vi "Auto State Machine.vi"   [LabVIEW 2013]
uses:
  typedefs/fg_typedef.ctl
  <vilib>/Rock Robotics/WPI/Solenoid/WPI_SolenoidValue.ctl
  typedefs/State Machine/singleUseSubstate.ctl
  typedefs/DevRef Type.ctl
  typedefs/State Machine/subStates.ctl
  typedefs/Vision/vision enable.ctl
  <vilib>/Rock Robotics/WPI/Solenoid/WPI_SolenoidSetEnum.vi
panel:
  # "A State Machine to Handle One or Two Ball Autonomous"
types:
  T1 = typedef "fg_typedef.ctl" = enum16{"Get", "Set"}
  T2 = typedef "WPI_SolenoidValue.ctl" = enum16{"Off", "On", "Forward", "Reverse"}
  T3 = typedef "singleUseSubstate.ctl" = enum16{"null", "wait", "shift high", "shift low", "extend shooter", "retract shooter", "latch", "unlatch", "end"}
  T4 = typedef "subStates.ctl" = enum16{"null", "wait", "driver control", "auto", "manual override", "hold position", "rotate", "pickup", "pass", "recover pass", "load", "goto shoot", "shoot high goal", "shoot low goal", "cancel arm", "cancel shooter", "end", "test"}
  T5 = typedef "vision enable.ctl" = enum16{"Enable", "Disable", "Stop"}
  T6 = typedef "DevRef Type.ctl" = enum16{"Shooter Solenoid", "Latch Solenoid", "Right Up Sensor", "Right Down Sensor", "Hold Sensor", "Arm Encoder"}
  T7 = typedef "WPI_EncoderDevRef.ctl" = cluster{"DevStatus":errorcluster, "EncoderIndex":T8, "CounterIndex":T9, "DistancePerCount":dbl, "Decoding Type":T10}
  T8 = typedef "FPGA_EncoderIdx.ctl" = enum8{"Enc 0", "Enc 1", "Enc 2", "Enc 3", "Invalid"}
  T9 = typedef "FPGA_CounterCtrSystemIndex.ctl" = enum8{"Ctr 0", "Ctr 1", "Ctr 2", "Ctr 3", "Ctr 4", "Ctr 5", "Ctr 6", "Ctr 7", "Invalid"}
  T10 = typedef "WPI_EncoderType.ctl" = enum16{"1x", "2x", "4x"}
  T11 = typedef "WPI_SolenoidDevRef.ctl" = cluster{"DevStatus":errorcluster, "Solenoid Module":T12, "Forward Solenoid Channel":T13, "Reverse Solenoid Channel":T13}
  T12 = typedef "FPGA_TypedefSolenoidModule.ctl" = enum16{"Solenoid Module 1", "Solenoid Module 2"}
  T13 = typedef "WPI_SolenoidChannel.ctl" = enum8{"Solenoid 1", "Solenoid 2", "Solenoid 3", "Solenoid 4", "Solenoid 5", "Solenoid 6", "Solenoid 7", "Solenoid 8", "Invalid"}
  T14 = typedef "WPI_DigitalInputDevRef.ctl" = cluster{"DevStatus":errorcluster, "DIO Channel":T15, "Digital Module":T16}
  T15 = typedef "FPGA_DIOChannel.ctl" = enum8{"DIO 1", "DIO 2", "DIO 3", "DIO 4", "DIO 5", "DIO 6", "DIO 7", "DIO 8", "DIO 9", "DIO 10", "DIO 11", "DIO 12", "DIO 13", "DIO 14", "Invalid"}
  T16 = typedef "FPGA_TypedefDigitalModule.ctl" = enum16{"Digital Module 1", "Digital Module 2"}
  T17 = typedef "vision data.ctl" = cluster{"x":dbl, "y":dbl, "area":dbl, "width":dbl, "height":dbl, "Hot Goal Present?":bool, "distance":dbl}
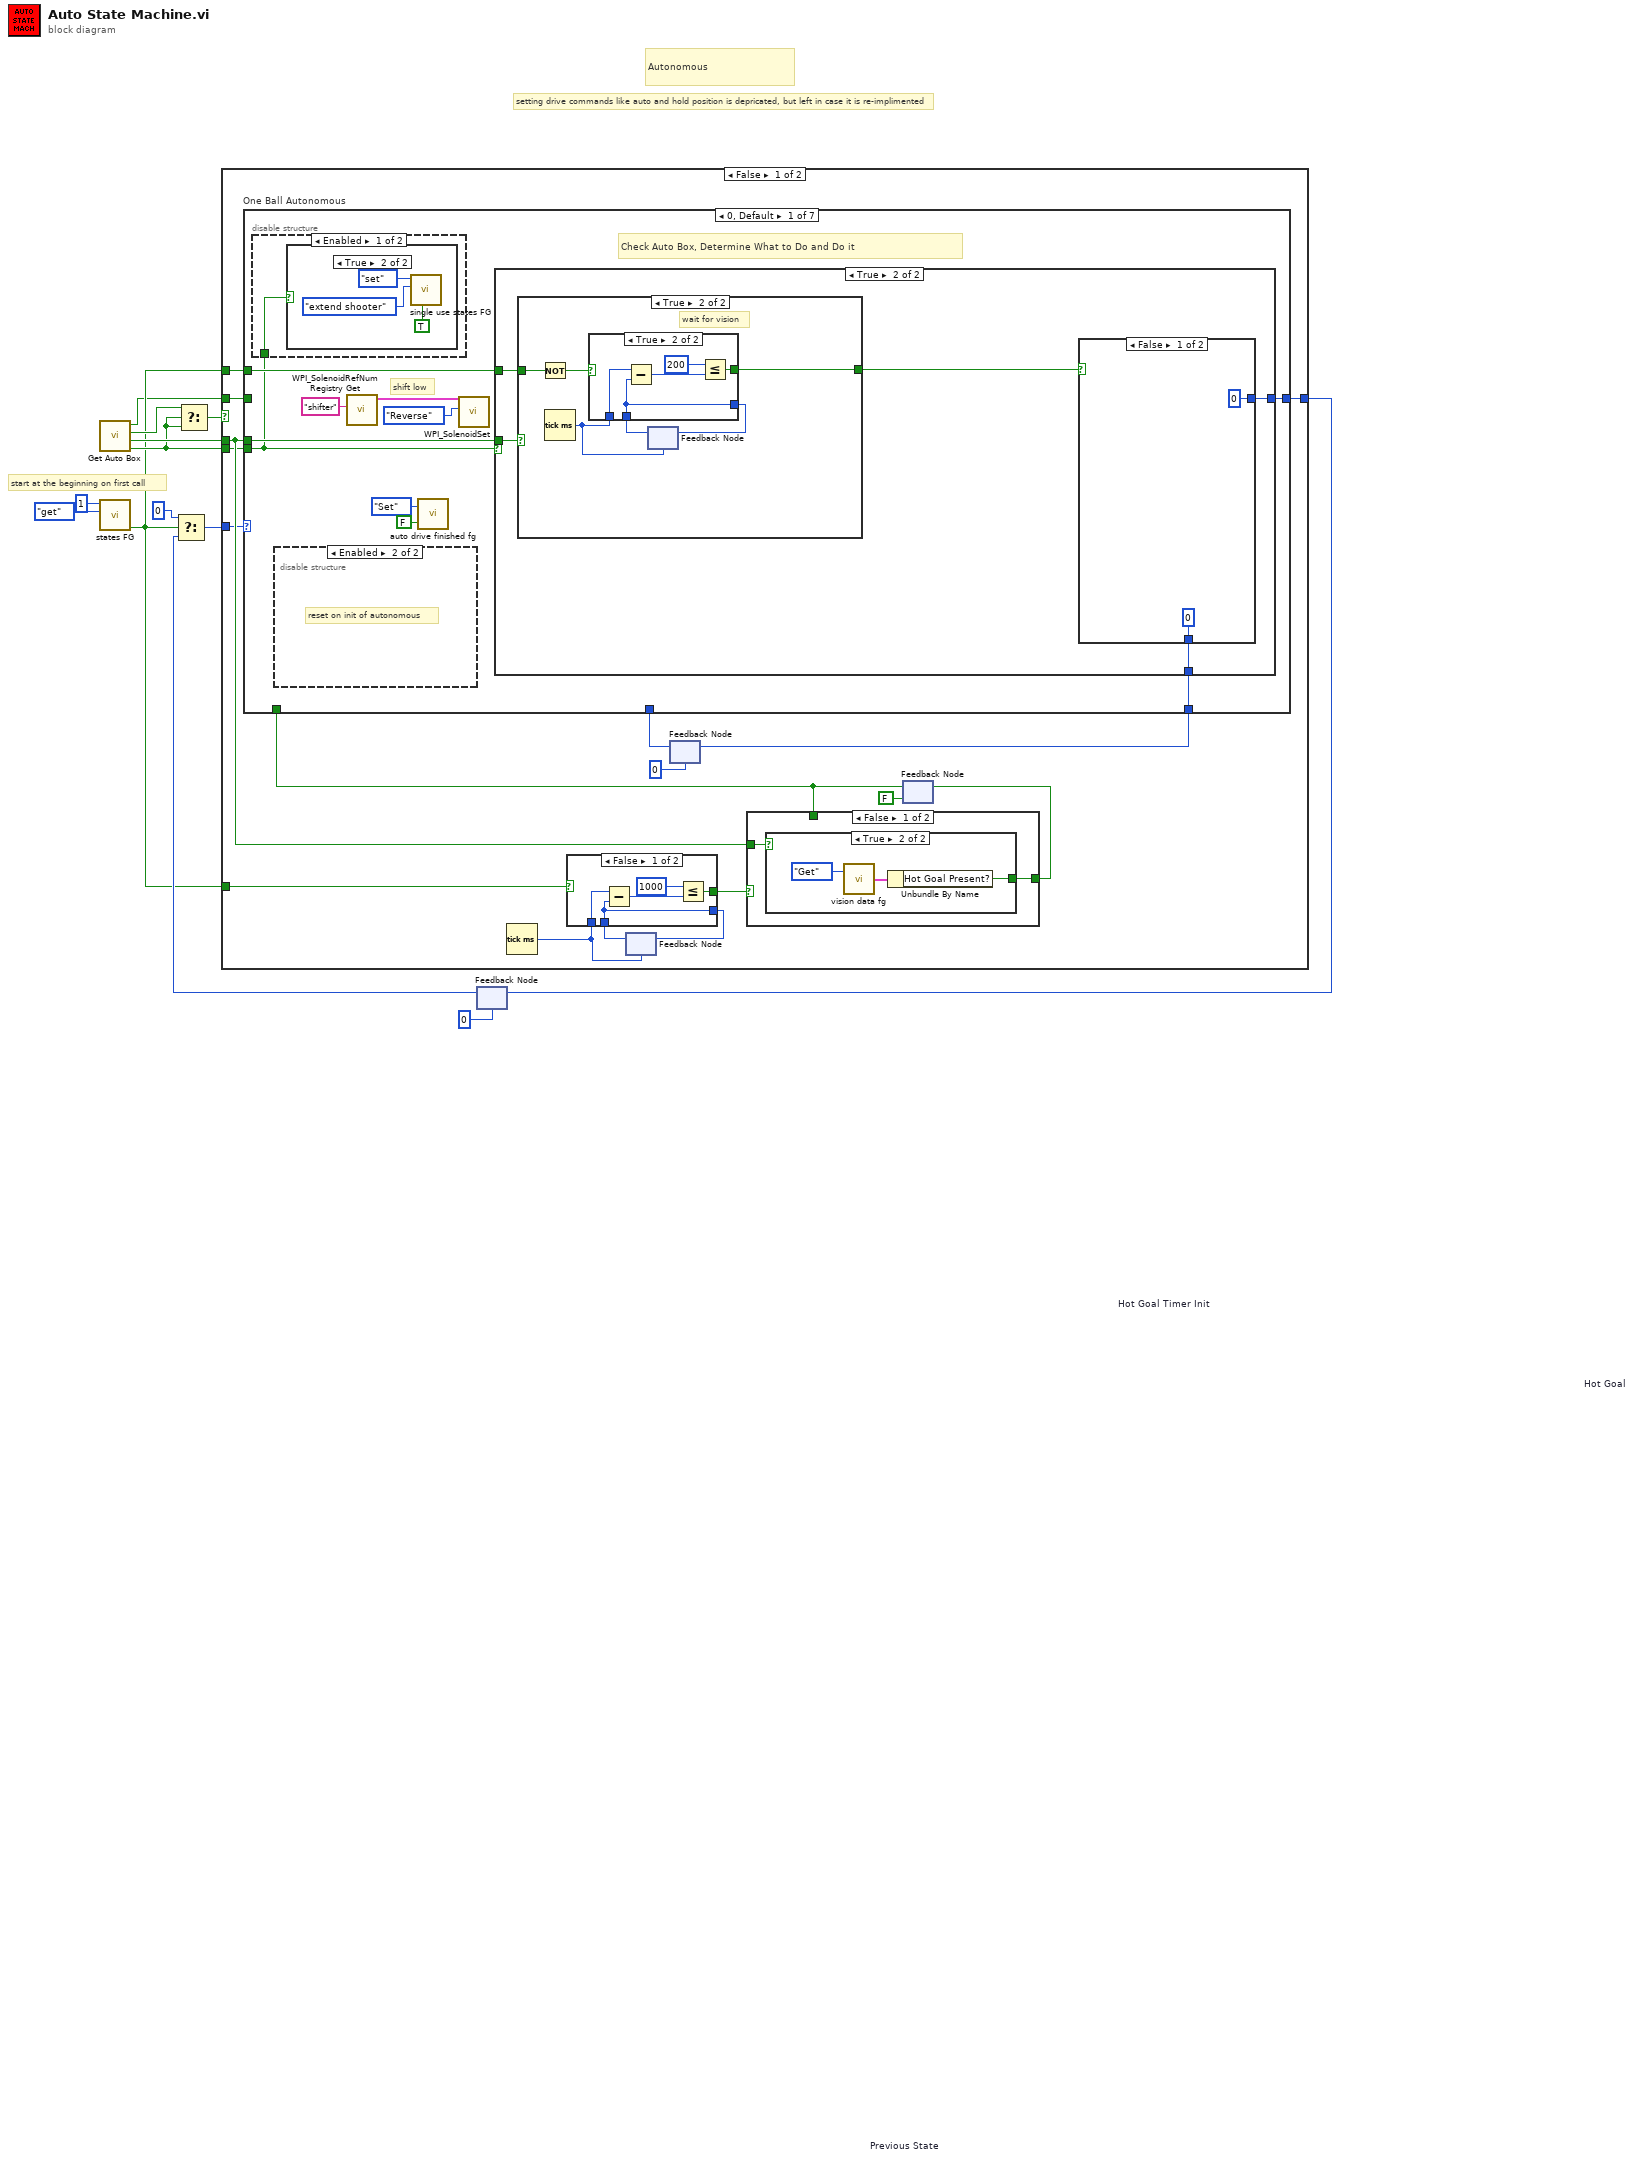
[diagram p0: block diagram]
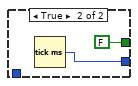
[diagram p2: hidden frame]
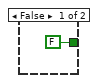
[diagram p3: hidden frame]
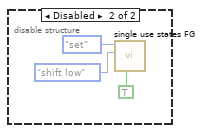
[diagram p6: hidden frame]
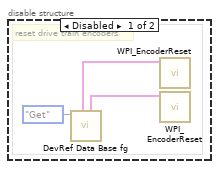
[diagram p7: hidden frame]
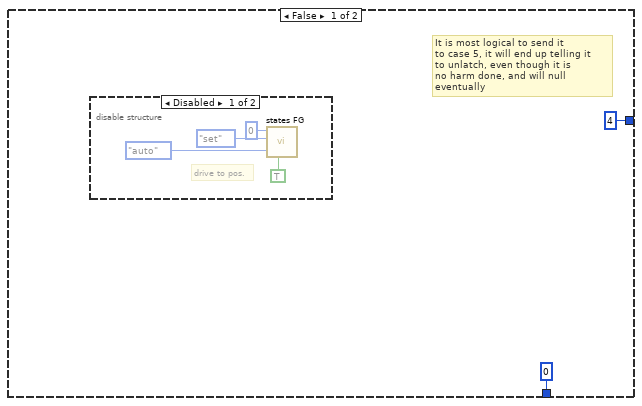
[diagram p8: hidden frame]
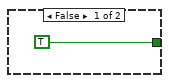
[diagram p10: hidden frame]
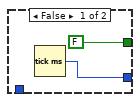
[diagram p11: hidden frame]
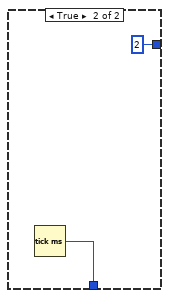
[diagram p12: hidden frame]
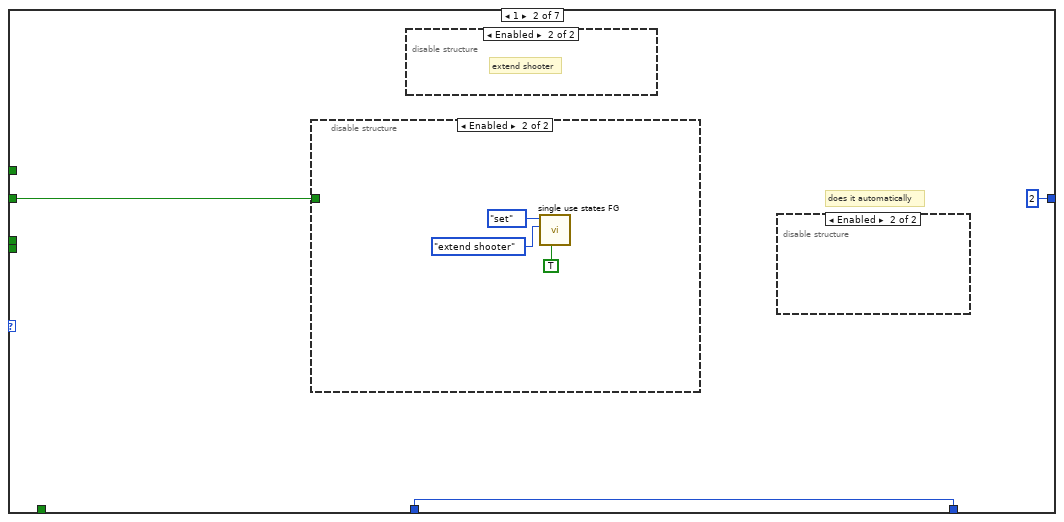
[diagram p13: hidden frame]
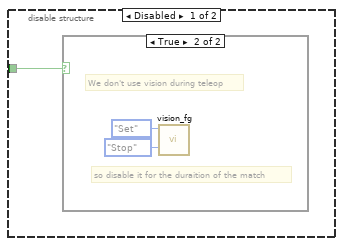
[diagram p15: hidden frame]
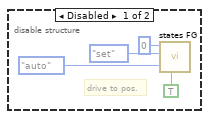
[diagram p17: hidden frame]
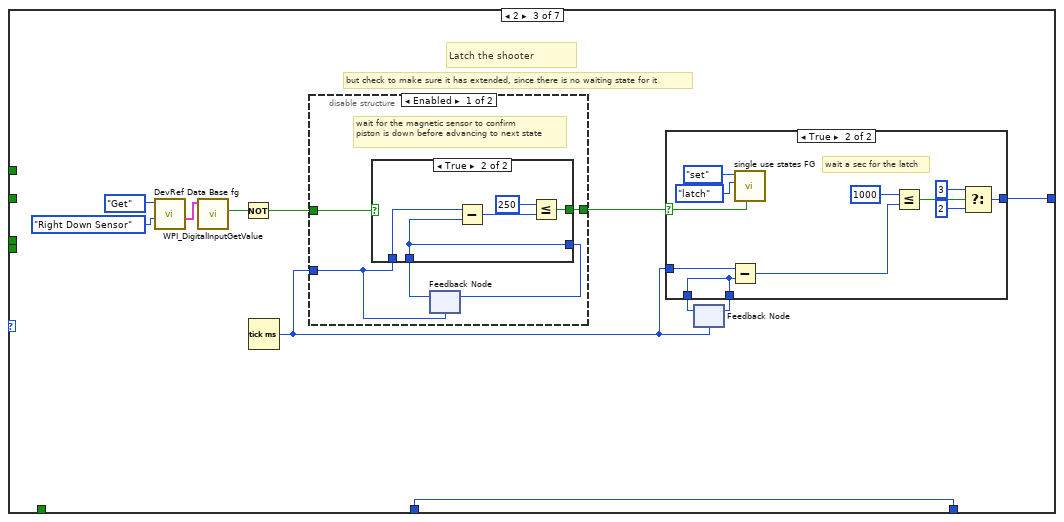
[diagram p18: hidden frame]
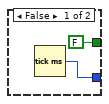
[diagram p19: hidden frame]
diagram:
  # "setting drive commands like auto and hold position is depricated, but left in case it is re-implimented"
  # "start at the beginning on first call"
  # "Autonomous"
  n1 = call "Get Auto Box.vi"() -> ("Shoot During Autonomous?"=w3:bool, "Use Hot Goal?"=w6:bool, "2 Ball Autonomous?"=w4:bool, "Disable Vison After Auto?"=w1:bool)
  n2 = call "states FG.vi"("menu (get)"=enum16{"set", "get"}."get", "Loop ID"=1) -> ("first call?"=w2:bool)  [unwired: 6 in, 3 out]
  n3 = Select(t=w4, s=w3, f=w3) -> (s? t:f=w5:bool)
  n4 = feedback #1 "Previous State"(u8 0) -> (w9:u8)
  n5 = Select(t=u8 0, s=w2, f=w9) -> (s? t:f=w11:u8)
  n6 = case shown="False" w5 {
    tunnel: w11 -> [w29 w236]
    tunnel: [w28 w229] -> w7
    tunnel: w2 -> [w26 w225]
    tunnel: w3 -> [w25 _]
    tunnel: w6 -> [w30 _]
    tunnel: w2 -> [w17 w233]
    tunnel: w1 -> [w23 _]
    frame False {
      n7 = Tick Count (ms)() -> (millisecond timer value=w15:u32)
      n8 = feedback #2(w15) -> (w20:u32)
      n9 = case shown="False" w17 {
        tunnel: [w32 w37] -> w19
        tunnel: w20 -> [w32 _]
        tunnel: [w33 FALSE] -> w18
        tunnel: w15 -> [w31 _]
        frame False {
          n10 = Subtract(x=w31, y=w32) -> (x-y=w35:u32)
          n11 = Less Or Equal?(x=u32 1000, y=w35) -> (x <= y?=w33:bool)
        }
        frame True {
          n12 = Tick Count (ms)() -> (millisecond timer value=w37:u32)
        }
      }
      n13 = feedback-in #2(w19) -> ()
      n14 = feedback #3 "Hot Goal Timer Init"(u32 0 ("millisecond timer value")) -> (w16:u32)
      n15 = feedback #4 "Hot Goal"(FALSE ("Hot Goal Present?")) -> (w14:bool)
      n16 = case "One Ball Autonomous" shown="0, Default" w29 {
        selector: w29 -> [_ _ _ _ w163 _ w222]
        tunnel: [w54 u8 2 ("t") w113 u8 4 ("t") w161 u8 6 ("t") w222] -> w28
        tunnel: w16 -> [_ w96 w107 w144 w151 w197 w205]
        tunnel: w26 -> [w53 _ _ _ _ _ _]
        tunnel: w25 -> [w51 _ _ _ w154 _ _]
        tunnel: w30 -> [w52 _ _ _ _ _ _]
        tunnel: [w50 w96 w107 w144 w151 w197 w205] -> w24
        tunnel: w23 -> [_ w94 _ _ _ _ w204]
        tunnel: w14 -> [_ _ _ _ w153 _ _]
        frame 0, Default {
          # "shift low"
          # "Check Auto Box, Determine What to Do and Do it"
          n17 = disable-structure shown="Enabled" {
            disable-tunnel: w51 -> [w55 _]
            frame Enabled {
              n18 = case shown="True" w55 {
                frame False {
                }
                frame True {
                  n19 = call "single use states FG.vi"("exit in"=TRUE, "substate"=singleUseSubstate."extend shooter", "menu (get)"=enum16{"set", "get"}."set") -> ()  [unwired: 5 in, 4 out]
                }
              }
            }
            frame Disabled {
              n20 = call "single use states FG.vi"("exit in"=TRUE, "substate"=singleUseSubstate."shift low", "menu (get)"=enum16{"set", "get"}."set") -> ()  [unwired: 5 in, 4 out]
            }
          }
          n21 = disable-structure shown="Enabled" {
            frame Disabled {
              # "reset drive train encoders"
              n22 = call "DevRef Data Base fg.vi"("Menu"=fg_typedef."Get") -> ("right drive encoder"=w62:T7, "left drive encoder"=w63:T7)  [unwired: 2 in, 7 out]
              n23 = call <vilib>:"WPI_EncoderReset.vi"("EncoderDevRef"=w63) -> ()  [unwired: 9 in, 2 out]
              n24 = call <vilib>:"WPI_EncoderReset.vi"("EncoderDevRef"=w62) -> ()  [unwired: 9 in, 2 out]
            }
            frame Enabled {
              # "reset on init of autonomous"
            }
          }
          n25 = call <vilib>:"WPI_SolenoidRefNum Registry Get.vi"("refnum name"="shifter") -> ("SolenoidDevRef"=w45:T11)  [unwired: 9 in, 1 out]
          n26 = call "auto drive finished fg.vi"("Done?"=FALSE, "Menu"=fg_typedef."Set") -> ()  [unwired: 1 out]
          n27 = call-poly <vilib>:"WPI_SolenoidSet.vi"("Value"=WPI_SolenoidValue."Reverse", "SolenoidDevRef"=w45) -> ()  [unwired: 8 in, 2 out]
          n28 = case shown="True" w51 {
            tunnel: [u8 4 ("f") w75] -> w54
            tunnel: w53 -> [_ w74]
            tunnel: w52 -> [_ w72]
            tunnel: [u32 0 ("millisecond timer value") w71] -> w50
            frame False {
              # "It is most logical to send it\nto case 5, it will end up telling it\nto unlatch, even though it is\nno harm done, and will null eventually"
              n29 = disable-structure shown="Disabled" {
                frame Disabled {
                  # "drive to pos."
                  n30 = call "states FG.vi"("exit in"=TRUE, "subState in"=subStates."auto", "menu (get)"=enum16{"set", "get"}."set", "Loop ID"=0) -> ()  [unwired: 4 in, 4 out]
                }
                frame Enabled {
                }
              }
            }
            frame True {
              n31 = case shown="True" w72 {
                tunnel: w74 -> [_ w82]
                tunnel: [TRUE w81] -> w73
                frame False {
                }
                frame True {
                  # "wait for vision"
                  n32 = Not(x=w82) -> (.not. x?=w77:bool)
                  n33 = Tick Count (ms)() -> (millisecond timer value=w80:u32)
                  n34 = feedback #5(w80) -> (w78:u32)
                  n35 = case shown="True" w77 {
                    tunnel: w80 -> [_ w87]
                    tunnel: [w84 w85] -> w79
                    tunnel: w78 -> [_ w85]
                    tunnel: [FALSE w86] -> w81
                    frame False {
                      n36 = Tick Count (ms)() -> (millisecond timer value=w84:u32)
                    }
                    frame True {
                      n37 = Subtract(x=w87, y=w85) -> (x-y=w89:u32)
                      n38 = Less Or Equal?(x=u32 200, y=w89) -> (x <= y?=w86:bool)
                    }
                  }
                  n39 = feedback-in #5(w79) -> ()
                }
              }
              n40 = case shown="False" w73 {
                tunnel: [u8 0 ("f") u8 2 ("f")] -> w75
                tunnel: [u32 0 ("millisecond timer value") w92] -> w71
                frame False {
                }
                frame True {
                  n41 = Tick Count (ms)() -> (millisecond timer value=w92:u32)
                }
              }
            }
          }
        }
        frame 1 {
          # "does it automatically"
          n42 = disable-structure shown="Enabled" {
            disable-tunnel: w94 -> [w97 _]
            frame Disabled {
              n43 = case shown="True" w97 {
                frame False {
                }
                frame True {
                  # "so disable it for the duraition of the match"
                  # "We don't use vision during teleop"
                  n44 = call "vision_fg.vi"("Action"=vision_enable."Stop", "Menu"=fg_typedef."Set" ("Enum")) -> ()  [unwired: 1 in, 2 out]
                }
              }
            }
            frame Enabled {
              n45 = call "single use states FG.vi"("exit in"=TRUE, "substate"=singleUseSubstate."extend shooter", "menu (get)"=enum16{"set", "get"}."set") -> ()  [unwired: 5 in, 4 out]
            }
          }
          n46 = disable-structure shown="Enabled" {
            frame Disabled {
              # "this has become completly unused now"
              # "Drive Up"
            }
            frame Enabled {
              # "extend shooter"
            }
          }
          n47 = disable-structure shown="Enabled" {
            frame Disabled {
              # "drive to pos."
              n48 = call "states FG.vi"("exit in"=TRUE, "subState in"=subStates."auto", "menu (get)"=enum16{"set", "get"}."set", "Loop ID"=0) -> ()  [unwired: 4 in, 4 out]
            }
            frame Enabled {
            }
          }
        }
        frame 2 {
          # "but check to make sure it has extended, since there is no waiting state for it"
          # "Latch the shooter"
          n49 = call "DevRef Data Base fg.vi"("DevRef to Get"=DevRef_Type."Right Down Sensor", "Menu"=fg_typedef."Get") -> ("Selected Sensor"=w117:T14)  [unwired: 1 in, 8 out]
          n50 = call <vilib>:"WPI_DigitalInputGetValue.vi"("DigitalInputDevRef"=w117) -> ("Value"=w116:bool)  [unwired: 8 in, 2 out]
          n51 = Not(x=w116) -> (.not. x?=w110:bool)
          n52 = Tick Count (ms)() -> (millisecond timer value=w109:u32)
          n53 = disable-structure shown="Enabled" {
            disable-tunnel: w110 -> [w122 w130]
            disable-tunnel: [w119 w130] -> w108
            disable-tunnel: w109 -> [w118 _]
            frame Enabled {
              # "wait for the magnetic sensor to confirm \npiston is down before advancing to next state"
              n54 = feedback #6(w118) -> (w120:u32)
              n55 = case shown="True" w122 {
                tunnel: w118 -> [_ w127]
                tunnel: [w124 w125] -> w121
                tunnel: w120 -> [_ w125]
                tunnel: [FALSE w126] -> w119
                frame False {
                  n56 = Tick Count (ms)() -> (millisecond timer value=w124:u32)
                }
                frame True {
                  n57 = Subtract(x=w127, y=w125) -> (x-y=w129:u32)
                  n58 = Less Or Equal?(x=u32 250, y=w129) -> (x <= y?=w126:bool)
                }
              }
              n59 = feedback-in #6(w121) -> ()
            }
            frame Disabled {
            }
          }
          n60 = feedback #7(w109) -> (w114:u32)
          n61 = case shown="True" w108 {
            selector: w108 -> [_ w139]
            tunnel: [w131 w141] -> w115
            tunnel: w114 -> [_ w141]
            tunnel: w109 -> [w131 w140]
            tunnel: [u8 2 ("f") w134] -> w113
            frame False {
              # "wait for the shooter"
            }
            frame True {
              # "wait a sec for the latch"
              n62 = Subtract(x=w140, y=w141) -> (x-y=w136:u32)
              n63 = call "single use states FG.vi"("exit in"=w139, "substate"=singleUseSubstate."latch", "menu (get)"=enum16{"set", "get"}."set") -> ()  [unwired: 5 in, 4 out]
              n64 = Less Or Equal?(x=u32 1000, y=w136) -> (x <= y?=w133:bool)
              n65 = Select(t=u8 3, s=w133, f=u8 2) -> (s? t:f=w134:u8)
            }
          }
          n66 = feedback-in #7(w115) -> ()
        }
        frame 3 {
          # "just go on, nothing to\nwait for"
          # "retract shooter"
          n67 = call "single use states FG.vi"("exit in"=TRUE, "substate"=singleUseSubstate."retract shooter", "menu (get)"=enum16{"set", "get"}."set") -> ()  [unwired: 5 in, 4 out]
        }
        frame 4 {
          # "depends on if shooting"
          # "at setpoint?"
          n68 = case shown="False" w153 {
            tunnel: w151 -> [w180 w186]
            tunnel: [w179 w185] -> w152
            frame True {
              # "get it first cycle after 3.5 seconds"
              n69 = Tick Count (ms)() -> (millisecond timer value=w181:u32)
              n70 = Subtract(x=w181, y=w180) -> (x-y=w183:u32)
              n71 = disable-structure shown="Disabled" {
                disable-tunnel: [_ FALSE ("Done")] -> w177
                frame Disabled {
                }
                frame Enabled {
                }
              }
              n72 = Less Or Equal?(x=u32 3500, y=w183) -> (x <= y?=w178:bool)
              n73 = Or(x=w178, y=w177) -> (x .or. y?=w179:bool)
            }
            frame False {
              # "wait 5.25 seconds for hot goal to switch"
              n74 = Tick Count (ms)() -> (millisecond timer value=w187:u32)
              n75 = Subtract(x=w187, y=w186) -> (x-y=w189:u32)
              n76 = Less Or Equal?(x=u32 5250, y=w189) -> (x <= y?=w185:bool)
            }
          }
          n77 = disable-structure shown="Enabled" {
            disable-tunnel: w151 -> [w166 _]
            frame Disabled {
              n78 = Tick Count (ms)() -> (millisecond timer value=w169:u32)
              n79 = Subtract(x=w169, y=w166) -> (x-y=w167:u32)
              n80 = Less Or Equal?(x=u32 4100, y=w167) -> (x <= y?=w165:bool)
              n81 = disable-structure shown="Enabled" {
                disable-tunnel: w165 -> [w171 _]
                disable-tunnel: fg_typedef."Set" ("Menu") -> [w170 _]
                frame Enabled {
                  n82 = case shown="True" w171 {
                    selector: w171 -> [_ w173]
                    tunnel: w170 -> [_ w172]
                    frame False {
                    }
                    frame True {
                      n83 = call "auto drive finished fg.vi"("Done?"=w173, "Menu"=w172) -> ()  [unwired: 1 out]
                      n84 = call "states FG.vi"("exit in"=w173, "subState in"=subStates."null" ("y"), "menu (get)"=enum16{"set", "get"}."set", "Loop ID"=0) -> ()  [unwired: 4 in, 4 out]
                    }
                  }
                }
                frame Disabled {
                }
              }
            }
            frame Enabled {
            }
          }
          n85 = call "DevRef Data Base fg.vi"("DevRef to Get"=DevRef_Type."Right Up Sensor", "Menu"=fg_typedef."Get") -> ("Selected Sensor"=w160:T14)  [unwired: 1 in, 8 out]
          n86 = call <vilib>:"WPI_DigitalInputGetValue.vi"("DigitalInputDevRef"=w160) -> ("Value"=w159:bool)  [unwired: 8 in, 2 out]
          n87 = Not(x=w159) -> (.not. x?=w156:bool)
          n88 = case shown="True" w156 {
            frame False {
            }
            frame True {
              # "incase we have problems,\nlet drivers trigger shoot after auto\nsince it is infact safe to shoot now"
              n89 = call "safe shoot error.vi"("Can Shoot Safely?"=TRUE, "Menu"=fg_typedef."Set") -> ()  [unwired: 1 out]
            }
          }
          n90 = call "auto drive finished fg.vi"("Menu"=fg_typedef."Get") -> ("Done"=w149:bool)  [unwired: 1 in]
          n91 = case shown="False" w154 {
            tunnel: w152 -> [_ w194]
            tunnel: w156 -> [_ w193]
            tunnel: w149 -> [w190 w192]
            tunnel: [w190 w191] -> w155
            frame False {
            }
            frame True {
              n92 = Compound Arithmetic op=AND(w194, w193, w192) -> (w191:bool)
            }
          }
          n93 = Select(t=u8 5, s=w155, f=w163) -> (s? t:f=w161:u8)
        }
        frame 5 {
          w200 = FALSE ("Can Shoot Safely?")
          w199 = fg_typedef."Set" ("Menu")
          # "unlatch shooter"
          # "SHOOT!!!"
          n94 = call "safe shoot error.vi"("Can Shoot Safely?"=w200, "Menu"=w199) -> ()  [unwired: 1 out]
          n95 = call "auto drive finished fg.vi"("Done?"=w200, "Menu"=w199) -> ()  [unwired: 1 out]
          n96 = call "single use states FG.vi"("exit in"=TRUE, "substate"=singleUseSubstate."unlatch", "menu (get)"=enum16{"set", "get"}."set") -> ()  [unwired: 5 in, 4 out]
        }
        frame 6 {
          # "null things"
          # "null all the things"
          n97 = case shown="True" w204 {
            frame False {
            }
            frame True {
              # "so disable it for the duraition of the match"
              # "We don't use vision during teleop"
              n98 = call "vision_fg.vi"("Action"=vision_enable."Stop", "Menu"=fg_typedef."Set" ("Enum")) -> ()  [unwired: 1 in, 2 out]
            }
          }
          n99 = call "states FG.vi"("exit in"=TRUE, "subState in"=subStates."null", "menu (get)"=enum16{"set", "get"}."set", "Loop ID"=0) -> ()  [unwired: 4 in, 4 out]
          n100 = call "states FG.vi"("exit in"=TRUE, "subState in"=subStates."null", "menu (get)"=enum16{"set", "get"}."set", "Loop ID"=1) -> ()  [unwired: 4 in, 4 out]
          n101 = call "states FG.vi"("exit in"=TRUE, "subState in"=subStates."null", "menu (get)"=enum16{"set", "get"}."set", "Loop ID"=2) -> ()  [unwired: 4 in, 4 out]
          n102 = call "states FG.vi"("exit in"=TRUE, "subState in"=subStates."null", "menu (get)"=enum16{"set", "get"}."set", "Loop ID"=3) -> ()  [unwired: 4 in, 4 out]
        }
      }
      n103 = feedback-in #3(w24) -> ()
      n104 = case shown="False" w18 {
        tunnel: [w39 w44] -> w21
        tunnel: w14 -> [_ w44]
        tunnel: w30 -> [w38 _]
        frame False {
          n105 = case shown="True" w38 {
            tunnel: [FALSE ("Hot Goal Present?") w43] -> w39
            frame False {
            }
            frame True {
              n106 = call "vision data fg.vi"("Menu"=fg_typedef."Get") -> ("Output"=w42:T17)  [unwired: 1 in]
              n107 = Unbundle By Name(w42) -> ("Hot Goal Present?"=w43:bool)
            }
          }
        }
        frame True {
        }
      }
      n108 = feedback-in #4(w21) -> ()
    }
    frame True {
      n109 = feedback #8 "Wait Timer Init"(u32 0 ("millisecond timer value")) -> (w226:u32)
      n110 = case "Two Ball Autonomous" shown="0, Default" w236 {
        selector: w236 -> [_ w313 _ w332 _ w366 _ _ w387 w425 _ w443]
        tunnel: [u8 1 ("t") w315 u8 3 ("t") w329 u8 5 ("t") w368 u8 7 ("t") u8 8 ("t") w388 w424 u8 11 ("t") w443] -> w229
        tunnel: [_ _ w323 w330 _ _ _ _ _ _ _ _] -> w227
        tunnel: w226 -> [_ _ _ w331 _ _ _ _ _ _ _ _]
        tunnel: w225 -> [w294 _ _ _ _ _ _ _ _ _ _ _]
        frame 0, Default {
          # "full reverse is belts in"
          # "belts on"
          # "up setpoint"
          # "put arm out"
          # "Arm Up, Belts In"
          # "reset drive train encoders"
          n111 = case shown="True" w294 {
            frame False {
            }
            frame True {
              # "so disable it for the duraition of the match"
              # "We don't use vision during teleop"
              n112 = call "vision_fg.vi"("Action"=vision_enable."Stop", "Menu"=fg_typedef."Set" ("Enum")) -> ()  [unwired: 1 in, 2 out]
            }
          }
          n113 = call "auto drive finished fg.vi"("Done?"=FALSE, "Menu"=fg_typedef."Set") -> ()  [unwired: 1 out]
          n114 = call "Arm Setpoint FG.vi"("Setpoint In"=55.0, "Menu"=fg_typedef."Set") -> ()  [unwired: 1 out]
          n115 = call "states FG.vi"("exit in"=TRUE, "subState in"=subStates."auto", "menu (get)"=enum16{"set", "get"}."set", "Loop ID"=3) -> ()  [unwired: 4 in, 4 out]
          n116 = call "Belt Speed FG.vi"("Speed In"=-1.0 ("Setpoint In"), "Menu"=fg_typedef."Set") -> ()  [unwired: 1 out]
          n117 = call "states FG.vi"("exit in"=TRUE, "subState in"=subStates."auto", "menu (get)"=enum16{"set", "get"}."set", "Loop ID"=2) -> ()  [unwired: 4 in, 4 out]
          n118 = call "DevRef Data Base fg.vi"("Menu"=fg_typedef."Get") -> ("right drive encoder"=w308:T7, "left drive encoder"=w309:T7)  [unwired: 2 in, 7 out]
          n119 = call <vilib>:"WPI_EncoderReset.vi"("EncoderDevRef"=w309) -> ()  [unwired: 9 in, 2 out]
          n120 = call <vilib>:"WPI_EncoderReset.vi"("EncoderDevRef"=w308) -> ()  [unwired: 9 in, 2 out]
        }
        frame 1 {
          # "Wait for Arm"
          n121 = call "DevRef Data Base fg.vi"("DevRef to Get"=DevRef_Type."Arm Encoder", "Menu"=fg_typedef."Get") -> ("Selected Encoder"=w322:T7)  [unwired: 1 in, 8 out]
          n122 = call <vilib>:"WPI_EncoderGet.vi"("EncoderDevRef"=w322) -> ("Distance"=w321:dbl)  [unwired: 5 in, 5 out]
          n123 = In Range and Coerce(upper limit=55.0, x=w321, lower limit=45.0) -> (In Range?=w314:bool)  [unwired: 1 out]
          n124 = Select(t=u8 2, s=w314, f=w313) -> (s? t:f=w315:u8)
        }
        frame 2 {
          # "drive to reverse position"
          n125 = Tick Count (ms)() -> (millisecond timer value=w323:u32)
          n126 = call "states FG.vi"("exit in"=TRUE, "subState in"=subStates."auto", "menu (get)"=enum16{"set", "get"}."set", "Loop ID"=0) -> ()  [unwired: 4 in, 4 out]
        }
        frame 3 {
          # "Wait for Ball"
          n127 = disable-structure shown="Enabled" {
            disable-tunnel: w332 -> [w334 w343]
            disable-tunnel: w331 -> [_ w345]
            disable-tunnel: [_ w345] -> w330
            disable-tunnel: [w333 w341] -> w329
            frame Disabled {
              n128 = call "DevRef Data Base fg.vi"("DevRef to Get"=DevRef_Type."Hold Sensor", "Menu"=fg_typedef."Get") -> ("Selected Sensor"=w338:T14)  [unwired: 1 in, 8 out]
              n129 = call <vilib>:"WPI_DigitalInputGetValue.vi"("DigitalInputDevRef"=w338) -> ("Value"=w340:bool)  [unwired: 8 in, 2 out]
              n130 = Not(x=w340) -> (.not. x?=w339:bool)
              n131 = Select(t=u8 4, s=w339, f=w334) -> (s? t:f=w333:u8)
            }
            frame Enabled {
              n132 = Tick Count (ms)() -> (millisecond timer value=w348:u32)
              n133 = Subtract(x=w348, y=w345) -> (x-y=w347:u32)
              n134 = Less Or Equal?(x=u32 1000, y=w347) -> (x <= y?=w344:bool)
              n135 = Select(t=u8 4, s=w344, f=w343) -> (s? t:f=w341:u8)
            }
          }
        }
        frame 4 {
          # "drive to forward position"
          # "arm rests on ball"
          # "reset fg"
          # "reset fg"
          # "Belts Off, Arm Hold Ball"
          n136 = call "states FG.vi"("exit in"=TRUE, "subState in"=subStates."auto", "menu (get)"=enum16{"set", "get"}."set", "Loop ID"=0) -> ()  [unwired: 4 in, 4 out]
          n137 = call "Belt Speed FG.vi"("Speed In"=0.0 ("Setpoint In"), "Menu"=fg_typedef."Set") -> ()  [unwired: 1 out]
          n138 = call "states FG.vi"("exit in"=TRUE, "subState in"=subStates."null", "menu (get)"=enum16{"set", "get"}."set", "Loop ID"=3) -> ()  [unwired: 4 in, 4 out]
          n139 = call "states FG.vi"("exit in"=TRUE, "subState in"=subStates."null", "menu (get)"=enum16{"set", "get"}."set", "Loop ID"=2) -> ()  [unwired: 4 in, 4 out]
          n140 = call "Arm Setpoint FG.vi"("Setpoint In"=0.0, "Menu"=fg_typedef."Set") -> ()  [unwired: 1 out]
        }
        frame 5 {
          w372 = fg_typedef."Get" ("Menu")
          # "Ready to Shoot 1st Ball?"
          n141 = call "safe shoot error.vi"("Menu"=w372) -> ("Can Shoot Safely?"=w371:bool)  [unwired: 1 in]
          n142 = call "auto drive finished fg.vi"("Menu"=w372) -> ("Done"=w370:bool)  [unwired: 1 in]
          n143 = And(x=w371, y=w370) -> (x .and. y?=w367:bool)
          n144 = Select(t=u8 6, s=w367, f=w366) -> (s? t:f=w368:u8)
        }
        frame 6 {
          w375 = FALSE ("Can Shoot Safely?")
          w374 = fg_typedef."Set" ("Menu")
          # "unlatch shooter"
          # "stop driving"
          n145 = call "states FG.vi"("exit in"=TRUE, "subState in"=subStates."hold position", "menu (get)"=enum16{"set", "get"}."set", "Loop ID"=0) -> ()  [unwired: 4 in, 4 out]
          n146 = call "safe shoot error.vi"("Can Shoot Safely?"=w375, "Menu"=w374) -> ()  [unwired: 1 out]
          n147 = call "auto drive finished fg.vi"("Done?"=w375, "Menu"=w374) -> ()  [unwired: 1 out]
          n148 = call "single use states FG.vi"("exit in"=TRUE, "substate"=singleUseSubstate."unlatch", "menu (get)"=enum16{"set", "get"}."set") -> ()  [unwired: 5 in, 4 out]
        }
        frame 7 {
          # "Cock again"
          # "extend shooter"
          n149 = call "single use states FG.vi"("exit in"=TRUE, "substate"=singleUseSubstate."extend shooter", "menu (get)"=enum16{"set", "get"}."set") -> ()  [unwired: 5 in, 4 out]
        }
        frame 8 {
          # "Wait to Latch Shooter, Then Latch"
          n150 = call "DevRef Data Base fg.vi"("DevRef to Get"=DevRef_Type."Right Down Sensor", "Menu"=fg_typedef."Get") -> ("Selected Sensor"=w390:T14)  [unwired: 1 in, 8 out]
          n151 = call <vilib>:"WPI_DigitalInputGetValue.vi"("DigitalInputDevRef"=w390) -> ("Value"=w389:bool)  [unwired: 8 in, 2 out]
          n152 = Tick Count (ms)() -> (millisecond timer value=w397:u32)
          n153 = Not(x=w389) -> (.not. x?=w393:bool)
          n154 = disable-structure shown="Enabled" {
            disable-tunnel: w393 -> [w415 w423]
            disable-tunnel: [w412 w423] -> w396
            disable-tunnel: w397 -> [w411 _]
            frame Enabled {
              # "wait for the magnetic sensor to confirm \npiston is down before advancing to next state"
              n155 = feedback #9(w411) -> (w413:u32)
              n156 = case shown="True" w415 {
                tunnel: w411 -> [_ w420]
                tunnel: [w417 w418] -> w414
                tunnel: w413 -> [_ w418]
                tunnel: [FALSE w419] -> w412
                frame False {
                  n157 = Tick Count (ms)() -> (millisecond timer value=w417:u32)
                }
                frame True {
                  n158 = Subtract(x=w420, y=w418) -> (x-y=w422:u32)
                  n159 = Less Or Equal?(x=u32 250, y=w422) -> (x <= y?=w419:bool)
                }
              }
              n160 = feedback-in #9(w414) -> ()
            }
            frame Disabled {
            }
          }
          n161 = feedback #10(w397) -> (w395:u32)
          n162 = case shown="True" w396 {
            selector: w396 -> [_ w406]
            tunnel: [w399 w408] -> w394
            tunnel: w395 -> [_ w408]
            tunnel: w397 -> [w399 w407]
            tunnel: [w398 w402] -> w388
            tunnel: w387 -> [w398 w400]
            frame False {
              # "wait for the shooter"
            }
            frame True {
              # "wait a sec for the latch"
              n163 = Subtract(x=w407, y=w408) -> (x-y=w403:u32)
              n164 = call "single use states FG.vi"("exit in"=w406, "substate"=singleUseSubstate."latch", "menu (get)"=enum16{"set", "get"}."set") -> ()  [unwired: 5 in, 4 out]
              n165 = Less Or Equal?(x=u32 1000, y=w403) -> (x <= y?=w401:bool)
              n166 = Select(t=u8 9, s=w401, f=w400) -> (s? t:f=w402:u8)
            }
          }
          n167 = feedback-in #10(w394) -> ()
        }
        frame 9 {
          # "Retract Shooter"
          # "retract shooter"
          n168 = call "single use states FG.vi"("exit in"=TRUE, "substate"=singleUseSubstate."retract shooter", "menu (get)"=enum16{"set", "get"}."set") -> ()  [unwired: 5 in, 4 out]
          n169 = call "DevRef Data Base fg.vi"("DevRef to Get"=DevRef_Type."Right Up Sensor", "Menu"=fg_typedef."Get") -> ("Selected Sensor"=w426:T14)  [unwired: 1 in, 8 out]
          n170 = call <vilib>:"WPI_DigitalInputGetValue.vi"("DigitalInputDevRef"=w426) -> ("Value"=w427:bool)  [unwired: 8 in, 2 out]
          n171 = Not(x=w427) -> (.not. x?=w431:bool)
          n172 = case shown="True" w431 {
            frame False {
            }
            frame True {
              # "incase we have problems,\nlet drivers trigger shoot after auto\nsince it is infact safe to shoot now"
              n173 = call "safe shoot error.vi"("Can Shoot Safely?"=TRUE, "Menu"=fg_typedef."Set") -> ()  [unwired: 1 out]
            }
          }
          n174 = Select(t=u8 10, s=w431, f=w425) -> (s? t:f=w424:u8)
        }
        frame 10 {
          w439 = FALSE ("Can Shoot Safely?")
          w438 = fg_typedef."Set" ("Menu")
          # "unlatch shooter"
          # "Shoot Second Ball"
          n175 = call "safe shoot error.vi"("Can Shoot Safely?"=w439, "Menu"=w438) -> ()  [unwired: 1 out]
          n176 = call "auto drive finished fg.vi"("Done?"=w439, "Menu"=w438) -> ()  [unwired: 1 out]
          n177 = call "single use states FG.vi"("exit in"=TRUE, "substate"=singleUseSubstate."unlatch", "menu (get)"=enum16{"set", "get"}."set") -> ()  [unwired: 5 in, 4 out]
        }
        frame 11 {
          # "Null Everything"
          # "null things"
          n178 = call "states FG.vi"("exit in"=TRUE, "subState in"=subStates."null", "menu (get)"=enum16{"set", "get"}."set", "Loop ID"=0) -> ()  [unwired: 4 in, 4 out]
          n179 = call "states FG.vi"("exit in"=TRUE, "subState in"=subStates."null", "menu (get)"=enum16{"set", "get"}."set", "Loop ID"=1) -> ()  [unwired: 4 in, 4 out]
          n180 = call "states FG.vi"("exit in"=TRUE, "subState in"=subStates."null", "menu (get)"=enum16{"set", "get"}."set", "Loop ID"=2) -> ()  [unwired: 4 in, 4 out]
          n181 = call "states FG.vi"("exit in"=TRUE, "subState in"=subStates."null", "menu (get)"=enum16{"set", "get"}."set", "Loop ID"=3) -> ()  [unwired: 4 in, 4 out]
        }
      }
      n182 = feedback-in #8(w227) -> ()
      n183 = feedback #11 "Previous State"(u8 0) -> (w231:u8)
      n184 = Select(t=u8 0, s=w233, f=w231) -> (s? t:f=w234:u8)
      n185 = case "Parallel Initial Pneumatics" shown="0, Default" w234 {
        selector: w234 -> [_ w241 w288 w291]
        tunnel: [u8 1 ("t") w244 w279 w291] -> w230
        frame 0, Default {
          # "Cock Shooter for Pre-Loaded Ball"
          # "extend shooter"
          n186 = call "single use states FG.vi"("exit in"=TRUE, "substate"=singleUseSubstate."extend shooter", "menu (get)"=enum16{"set", "get"}."set") -> ()  [unwired: 5 in, 4 out]
        }
        frame 1 {
          # "Wait to Latch Shooter, Then Latch"
          n187 = call "DevRef Data Base fg.vi"("DevRef to Get"=DevRef_Type."Right Down Sensor", "Menu"=fg_typedef."Get") -> ("Selected Sensor"=w250:T14)  [unwired: 1 in, 8 out]
          n188 = call <vilib>:"WPI_DigitalInputGetValue.vi"("DigitalInputDevRef"=w250) -> ("Value"=w251:bool)  [unwired: 8 in, 2 out]
          n189 = Tick Count (ms)() -> (millisecond timer value=w242:u32)
          n190 = Not(x=w251) -> (.not. x?=w247:bool)
          n191 = disable-structure shown="Enabled" {
            disable-tunnel: w247 -> [w269 w277]
            disable-tunnel: [w266 w277] -> w243
            disable-tunnel: w242 -> [w265 _]
            frame Enabled {
              # "wait for the magnetic sensor to confirm \npiston is down before advancing to next state"
              n192 = feedback #12(w265) -> (w267:u32)
              n193 = case shown="True" w269 {
                tunnel: w265 -> [_ w274]
                tunnel: [w271 w272] -> w268
                tunnel: w267 -> [_ w272]
                tunnel: [FALSE w273] -> w266
                frame False {
                  n194 = Tick Count (ms)() -> (millisecond timer value=w271:u32)
                }
                frame True {
                  n195 = Subtract(x=w274, y=w272) -> (x-y=w276:u32)
                  n196 = Less Or Equal?(x=u32 250, y=w276) -> (x <= y?=w273:bool)
                }
              }
              n197 = feedback-in #12(w268) -> ()
            }
            frame Disabled {
            }
          }
          n198 = feedback #13(w242) -> (w245:u32)
          n199 = case shown="True" w243 {
            selector: w243 -> [_ w260]
            tunnel: [w253 w262] -> w246
            tunnel: w245 -> [_ w262]
            tunnel: w242 -> [w253 w261]
            tunnel: [w252 w256] -> w244
            tunnel: w241 -> [w252 w254]
            frame False {
              # "wait for the shooter"
            }
            frame True {
              # "wait a sec for the latch"
              n200 = Subtract(x=w261, y=w262) -> (x-y=w257:u32)
              n201 = call "single use states FG.vi"("exit in"=w260, "substate"=singleUseSubstate."latch", "menu (get)"=enum16{"set", "get"}."set") -> ()  [unwired: 5 in, 4 out]
              n202 = Less Or Equal?(x=u32 1000, y=w257) -> (x <= y?=w255:bool)
              n203 = Select(t=u8 2, s=w255, f=w254) -> (s? t:f=w256:u8)
            }
          }
          n204 = feedback-in #13(w246) -> ()
        }
        frame 2 {
          # "retract shooter"
          # "Retract Shooter"
          n205 = call "single use states FG.vi"("exit in"=TRUE, "substate"=singleUseSubstate."retract shooter", "menu (get)"=enum16{"set", "get"}."set") -> ()  [unwired: 5 in, 4 out]
          n206 = call "DevRef Data Base fg.vi"("DevRef to Get"=DevRef_Type."Right Up Sensor", "Menu"=fg_typedef."Get") -> ("Selected Sensor"=w284:T14)  [unwired: 1 in, 8 out]
          n207 = call <vilib>:"WPI_DigitalInputGetValue.vi"("DigitalInputDevRef"=w284) -> ("Value"=w283:bool)  [unwired: 8 in, 2 out]
          n208 = Not(x=w283) -> (.not. x?=w278:bool)
          n209 = case shown="True" w278 {
            frame False {
            }
            frame True {
              # "incase we have problems,\nlet drivers trigger shoot after auto\nsince it is infact safe to shoot now"
              n210 = call "safe shoot error.vi"("Can Shoot Safely?"=TRUE, "Menu"=fg_typedef."Set") -> ()  [unwired: 1 out]
            }
          }
          n211 = Select(t=u8 3, s=w278, f=w288) -> (s? t:f=w279:u8)
        }
        frame 3 {
        }
      }
      n212 = feedback-in #11(w230) -> ()
    }
  }
  n213 = feedback-in #1(w7) -> ()
